vi "main.vi"() -> ()   [LabVIEW 2023]
uses:
  <vilib>/Hampel Software Engineering/Git API/Git API/GIT-api.lvclass
  <vilib>/Utility/miscctls.llb/LVComboBoxStrsAndValuesArrayTypeDef.ctl
  <vilib>/Hampel Software Engineering/Git API/Git API/GIT-api.lvclass/GIT-api.ctl
  <userlib>/_OpenG.lib/file/file.llb/openg_file.lvlib
panel:
  in  "OK":bool
  in  "Repo Url":string="https://github.com/keerthivarman-nageshwaran/LabVIEWGitTool.git"
  in  "Tree":string(tree)
  in  "To":string(combo)
  in  "From":string(combo)
  in  "Diff Tree":string(tree)
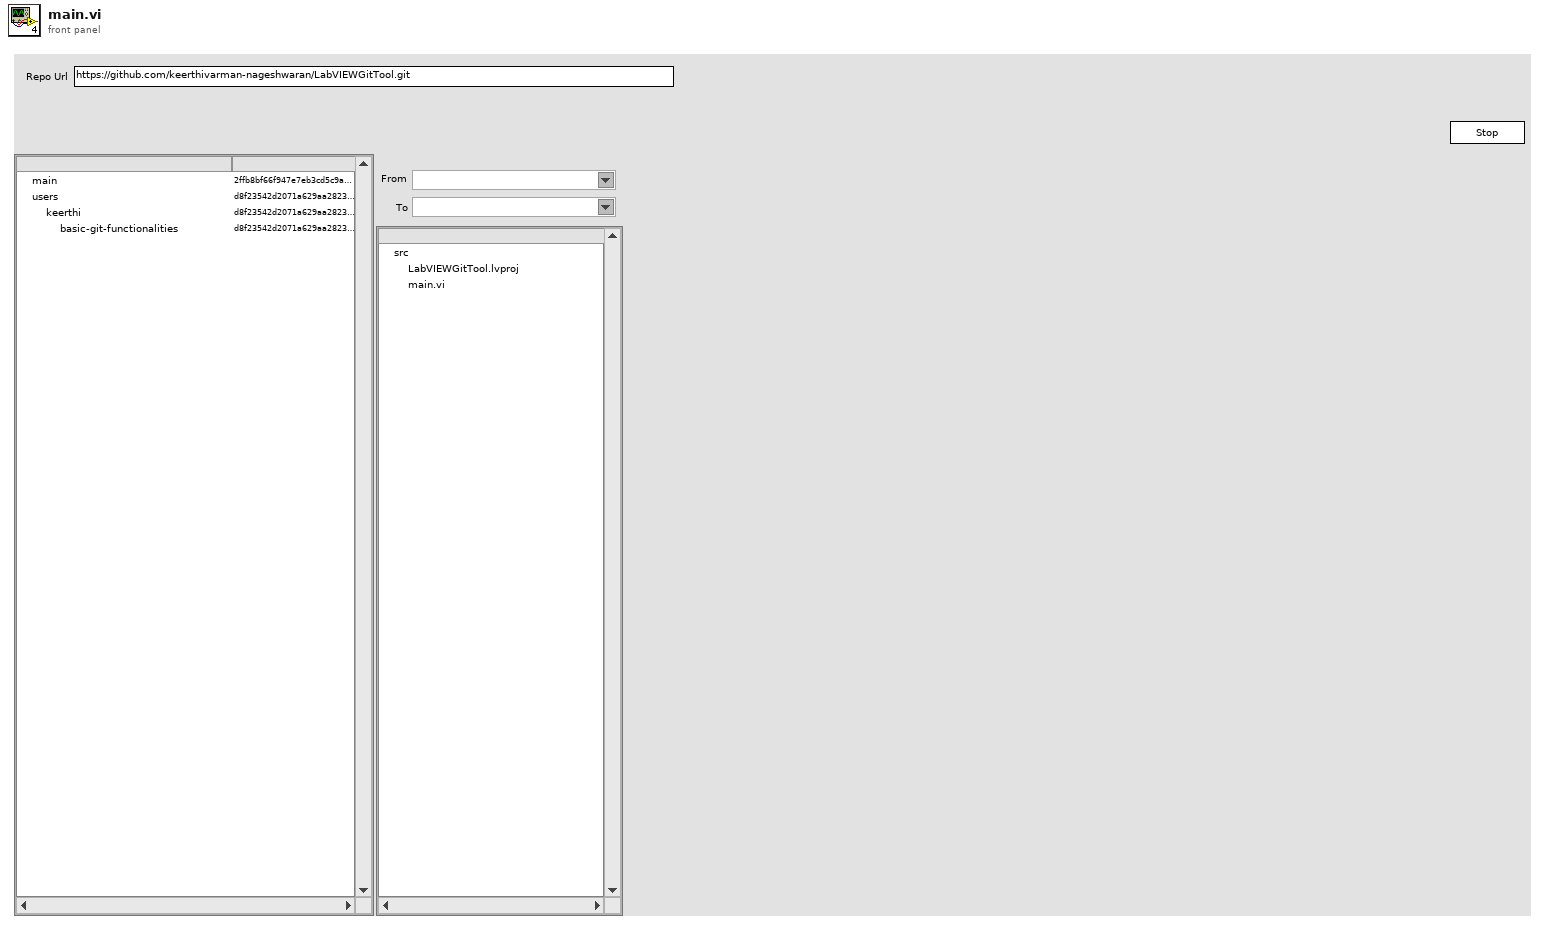
[diagram p1: front panel]
types:
  T1 = cluster{"Core":cluster{"Current VI Reference":refnum<vi>, "Close Panel on Exit?":bool}, "Git":cluster{"Local Repo Path":path, "Repo Url":string, "Temp Path":path, "git-api":refnum<class "GIT-api.lvclass">, "Branches":cluster{"Name":string, "Hash":string}[]}, "UI":cluster{"Tree":refnum<vi>, "Diff Tree":refnum<vi>}, "Diff":cluster{"To":string, "From":string, "Files":string[]}}
  T2 = enum32{"Invalid", "Standard", "Closed", "Hidden", "Minimized", "Maximized"}
  T3 = enum32{"invalid app kind", "Development System", "Run Time System", "Student Edition", "Embedded LabVIEW", "Evaluation", "Custom"}
  T4 = typedef "LVComboBoxStrsAndValuesArrayTypeDef.ctl" = cluster{"String":string, "Value":string}[]
  T5 = cluster{"Current VI Reference":refnum<vi>, "Close Panel on Exit?":bool}
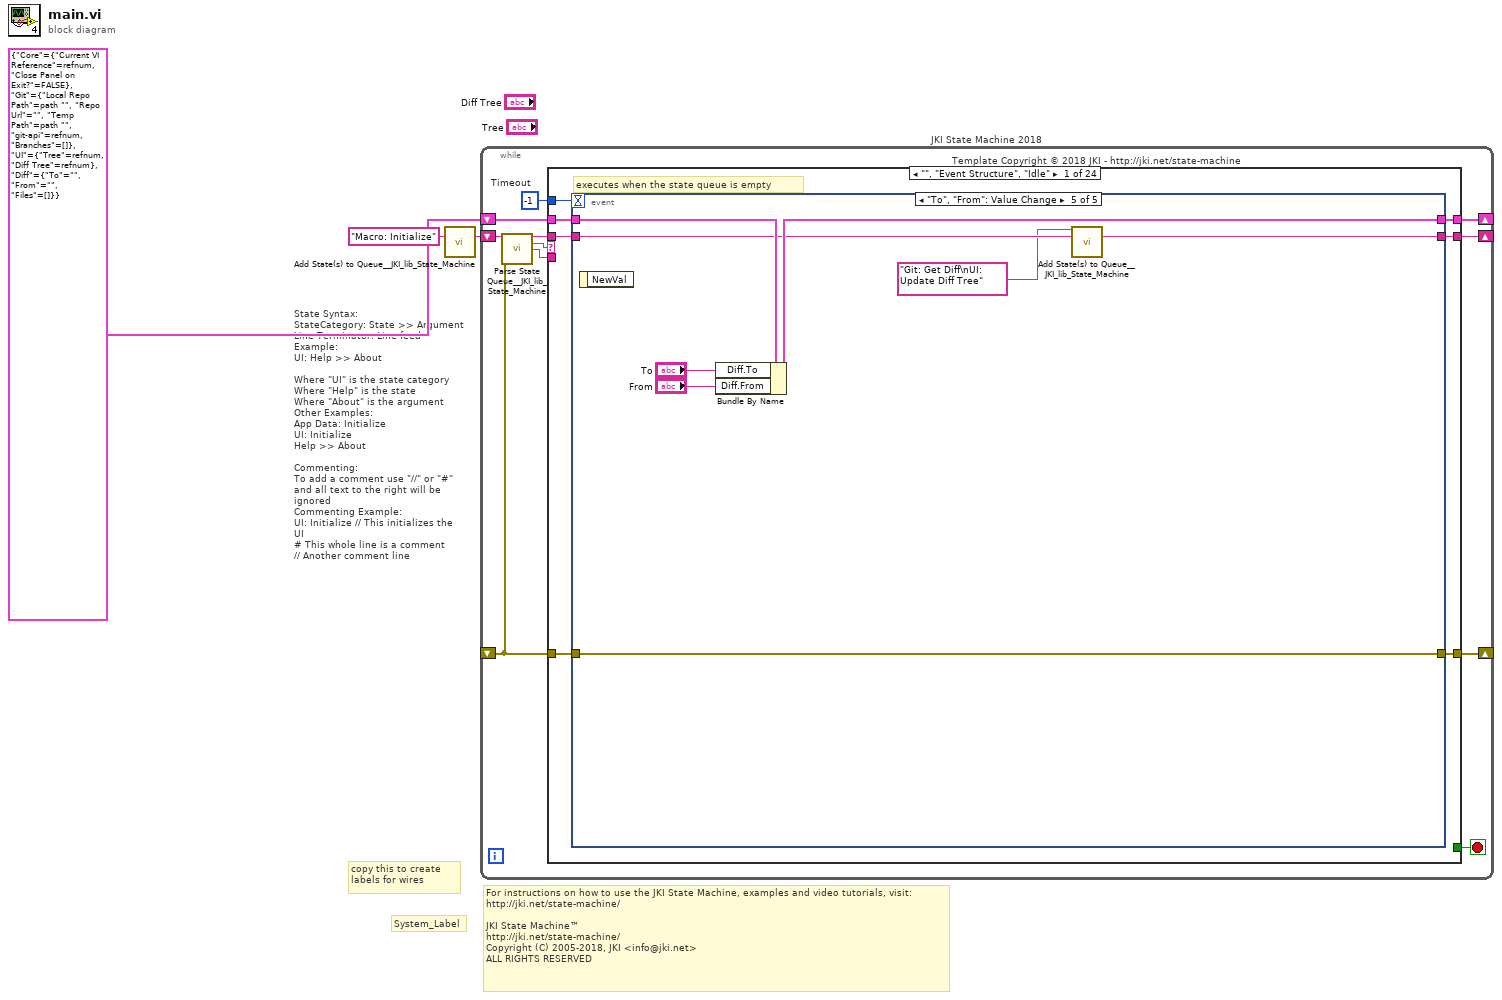
[diagram p0: block diagram]
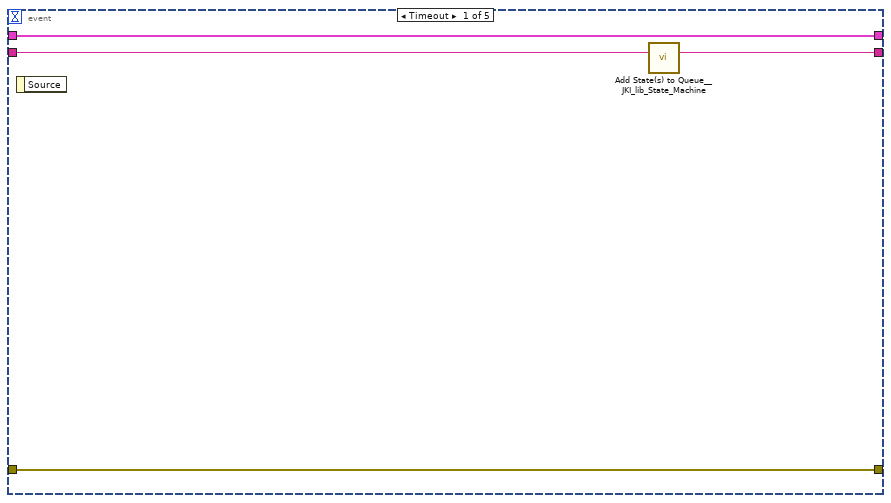
[diagram p2: hidden frame]
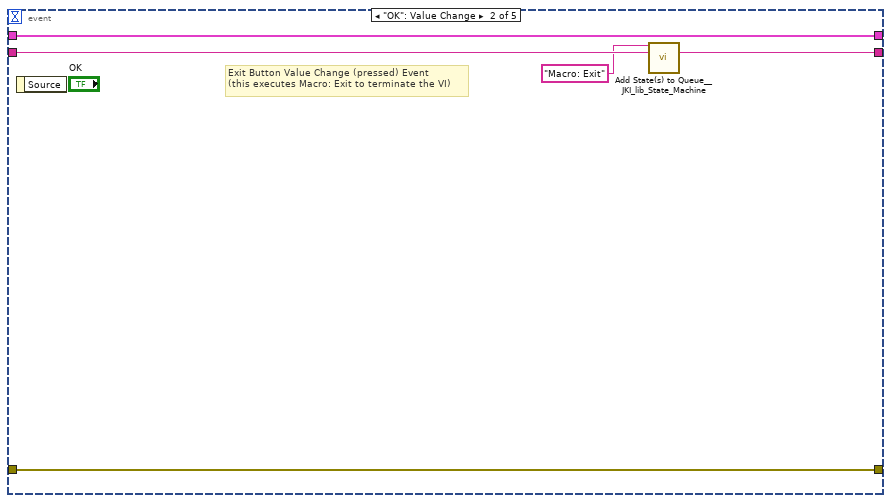
[diagram p3: hidden frame]
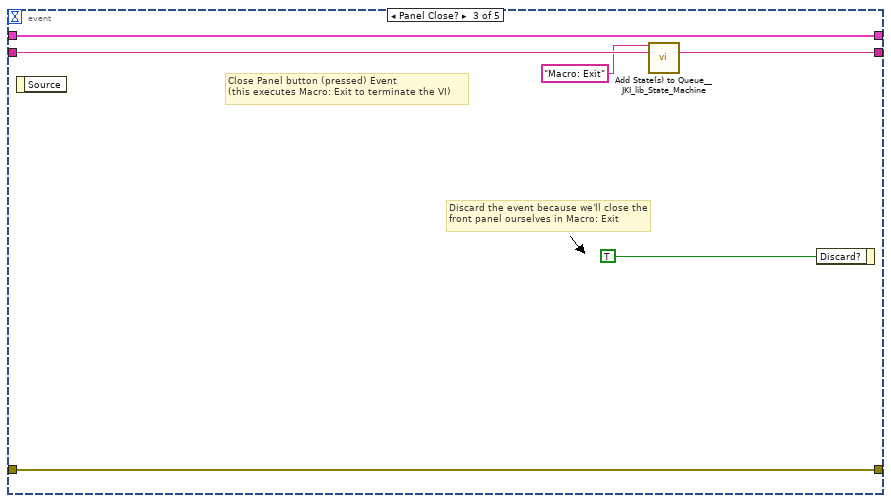
[diagram p4: hidden frame]
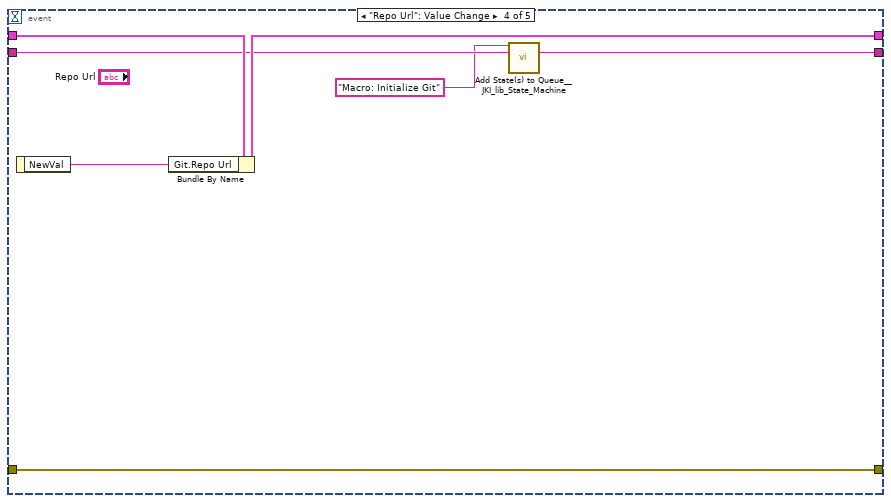
[diagram p5: hidden frame]
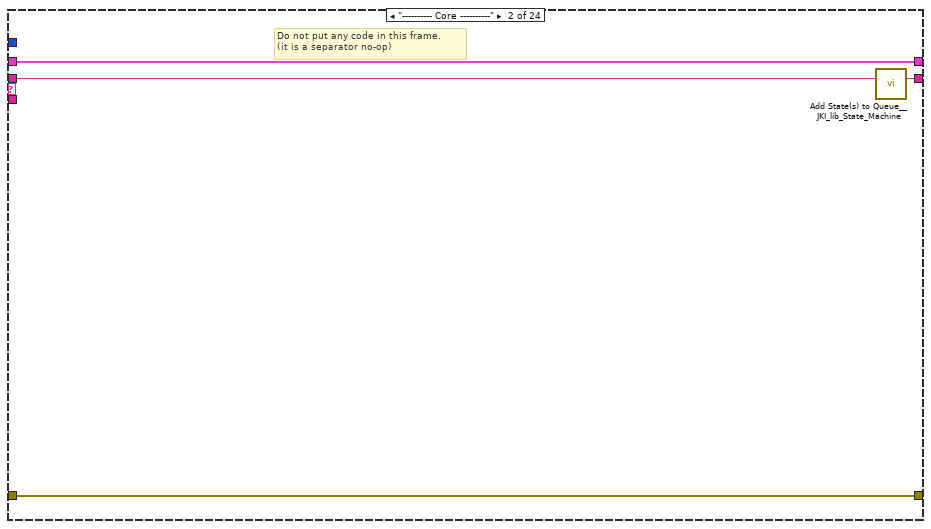
[diagram p6: hidden frame]
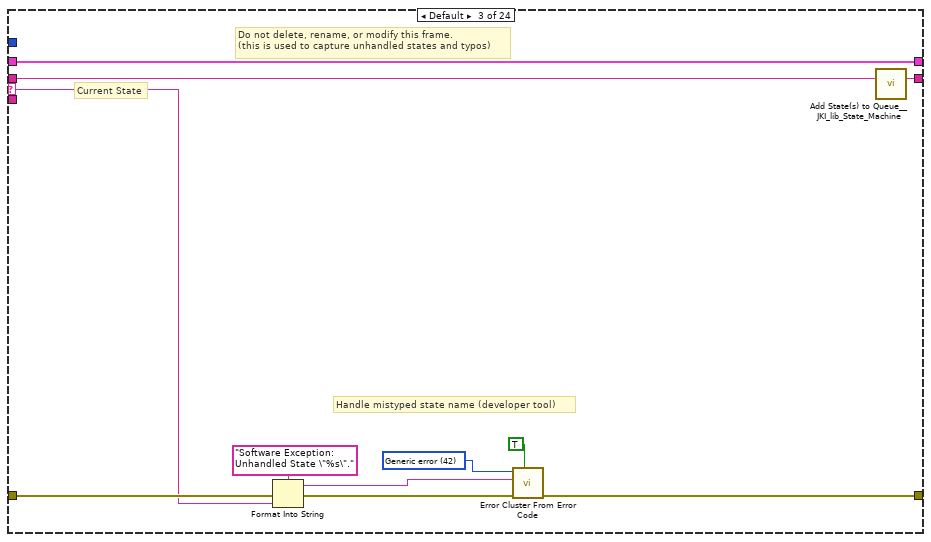
[diagram p7: hidden frame]
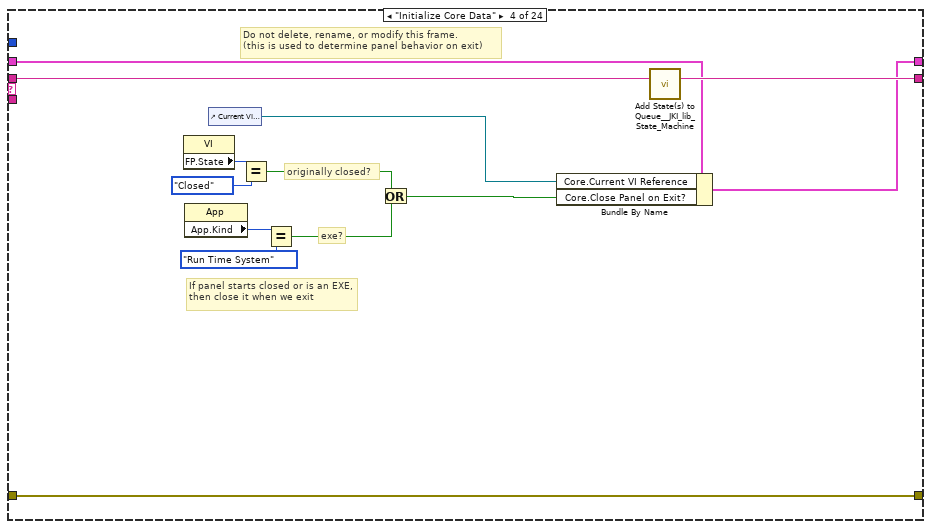
[diagram p8: hidden frame]
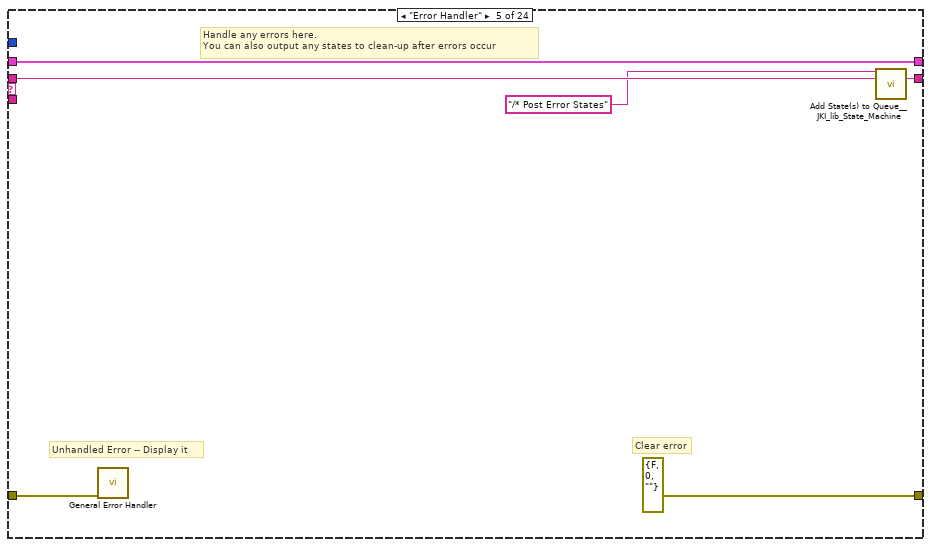
[diagram p9: hidden frame]
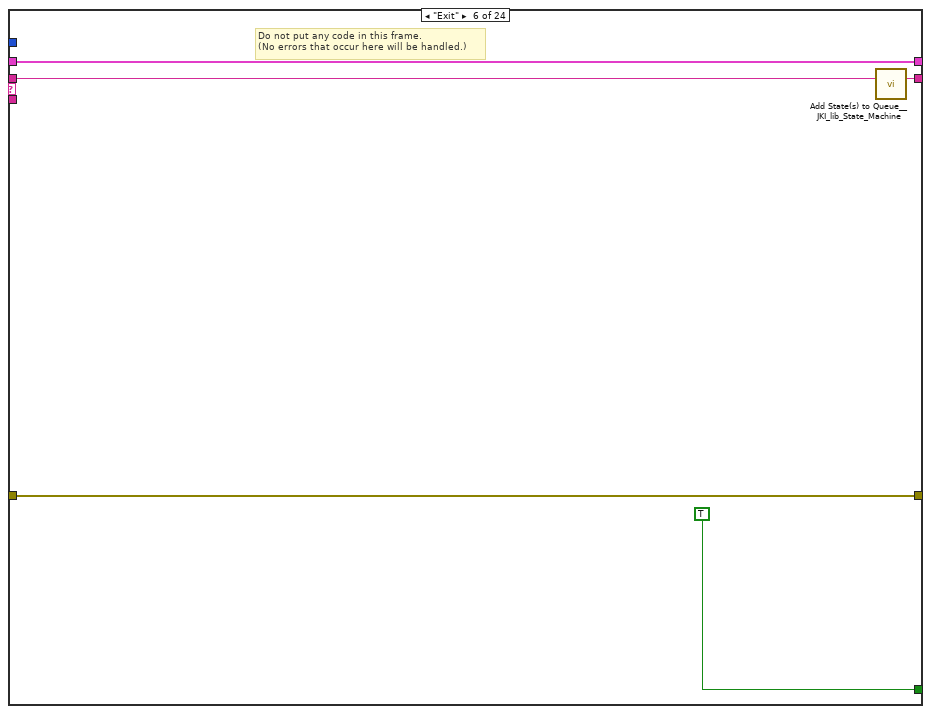
[diagram p10: hidden frame]
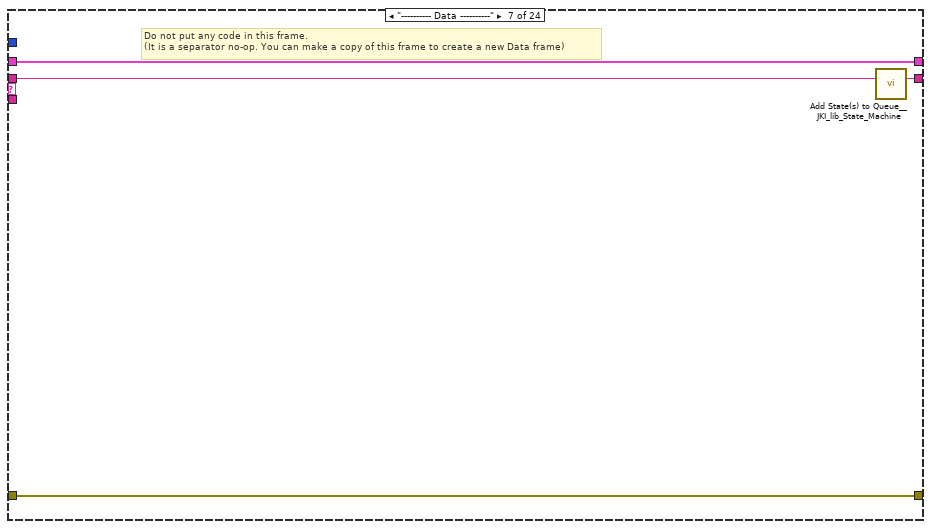
[diagram p11: hidden frame]
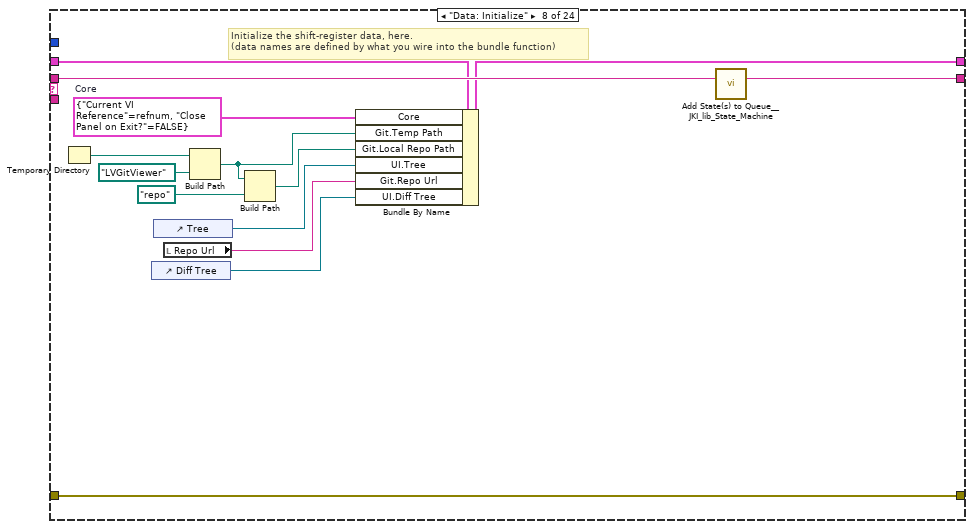
[diagram p12: hidden frame]
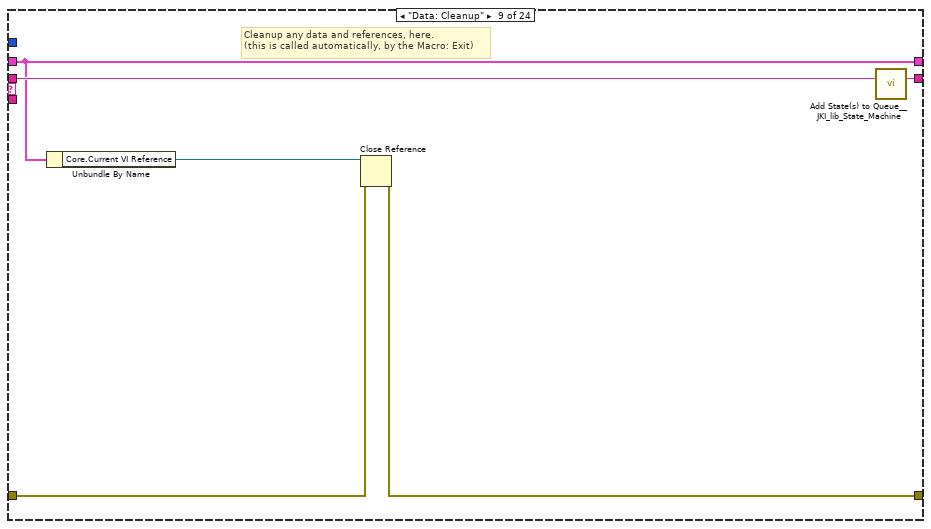
[diagram p13: hidden frame]
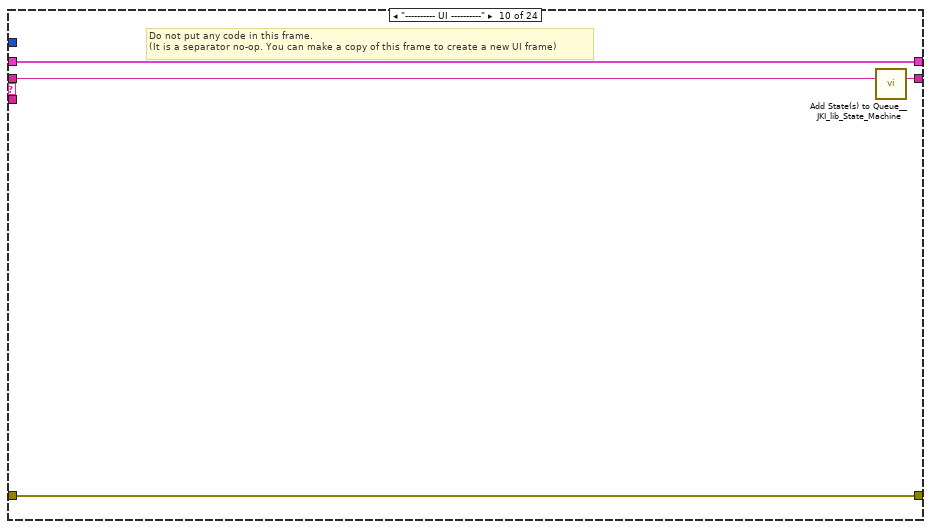
[diagram p14: hidden frame]
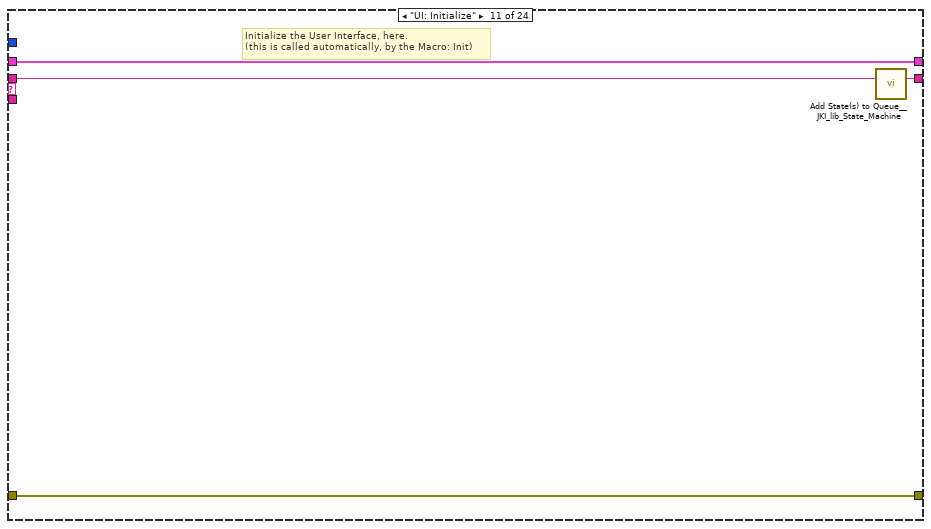
[diagram p15: hidden frame]
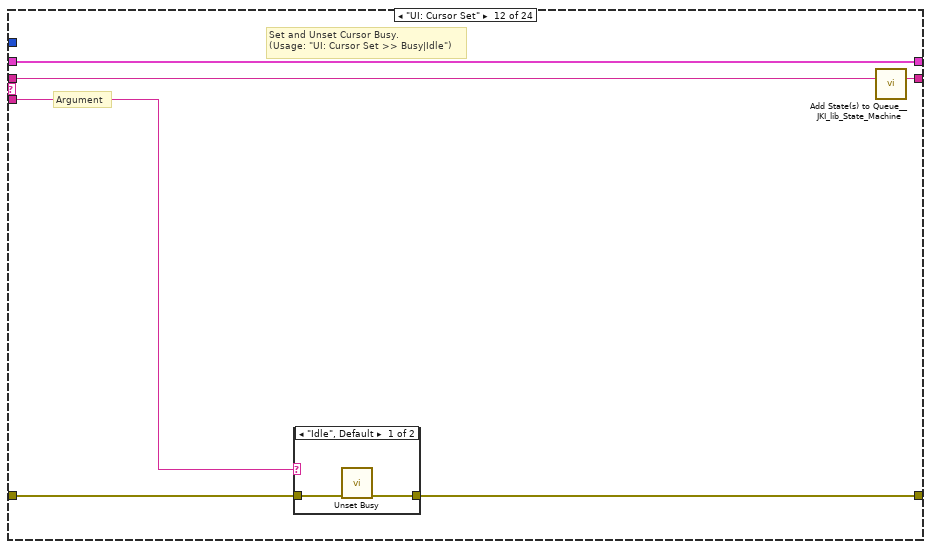
[diagram p16: hidden frame]
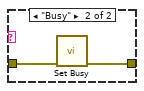
[diagram p17: hidden frame]
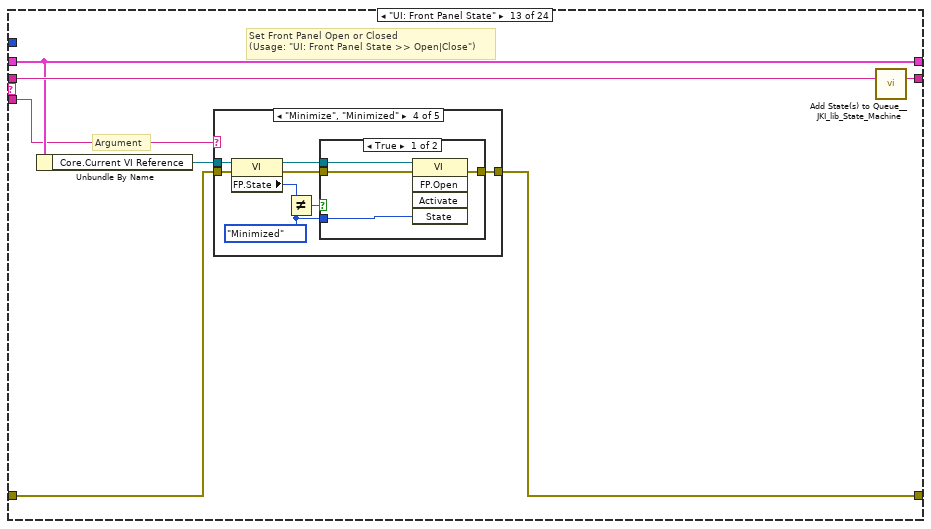
[diagram p18: hidden frame]
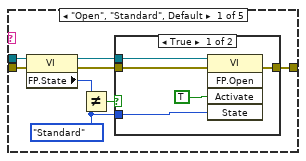
[diagram p19: hidden frame]
diagram:
  # "For instructions on how to use the JKI State Machine, examples and video tutorials, visit:\nhttp://jki.net/state-machine/\n\nJKI State Machine™\nhttp://jki.net/state-machine/\nCopyright (C) 2005-2018, JKI <info@jki.net>\nALL RIGHTS RESERVED"
  # "State Syntax:\nStateCategory: State >> Argument\nLine Terminator: Line feed\nExample:\nUI: Help >> About\n\nWhere \"UI\" is the state category\nWhere \"Help\" is the state\nWhere \"About\" is the argument\nOther Examples:\nApp Data: Initialize\nUI: Initialize\nHelp >> About\n\nCommenting:\nTo add a comment use \"//\" or \"#\" and all text to the right will be ignored\nCommenting Example:\nUI: Initialize // This initializes the UI\n# This whole line is a comment\n// Another comment line"
  # "copy this to create labels for wires"
  # "System_Label"
  n1 = call <vilib>:"Add State(s) to Queue__JKI_lib_State_Machine.vi"("State(s) in (\"\")"="Macro: Initialize") -> ("States Out"=w3:string)  [unwired: 14 in]
  n2 = while "JKI State Machine 2018" {
    shift-right: [w7] -> _
    shift-left: T1 {"Core"={"Current VI Reference"=refnum, "Close Panel on Exit?"=FALSE}, "Git"={"Local Repo Path"=path "", "Repo Url"="", "Temp Path"=path "", "git-api"=refnum, "Branches"=[]}, "UI"={"Tree"=refnum, "Diff Tree"=refnum}, "Diff"={"To"="", "From"="", "Files"=[]}} -> [w6]
    shift-right: [w10] -> _
    shift-left: _ -> [w4]
    shift-right: [w9] -> _
    shift-left: w3 -> [w11]
    stop <- w8 stop-if-true
    w5 = -1  # Timeout
    # "Template Copyright © 2018 JKI - http://jki.net/state-machine"
    n3 = call <vilib>:"Parse State Queue__JKI_lib_State_Machine.vi"("State Queue"=w11, "Error In (no error)"=w4) -> ("Remaining States"=w13:string, "Current State"=w14:string, "Arguments"=w12:string)  [unwired: 11 in]
    n4 = case shown="\"\", \"Event Structure\", \"Idle\"" w14 {
      selector: w14 -> [_ _ w56 _ _ _ _ _ _ _ _ _ _ _ _ _ _ _ _ _ _ _ _ _]
      tunnel: w13 -> [w21 w55 w60 w79 w85 w90 w94 w108 w114 w118 w122 w128 w139 w216 w231 w248 w254 w259 w269 w274 w278 w289 w316 w335]
      tunnel: w12 -> [_ _ _ _ _ _ _ _ _ _ _ w123 w133 _ _ _ _ _ _ _ _ _ _ _]
      tunnel: w6 -> [w19 w52 w58 w72 w82 w88 w91 w104 w109 w115 w120 w126 w135 w212 w229 w244 w251 w256 w266 w271 w275 w287 w314 w333]
      tunnel: [w18 w53 w62 w76 errorcluster {"status"=FALSE, "code"=0, "source"=""} ("error out") w87 w92 w103 w110 w116 w119 w124 w136 w214 w224 w246 w252 w257 w267 w272 w276 w284 w309 w331] -> w10
      tunnel: w4 -> [w17 w53 w61 w76 w81 w87 w92 w103 w111 w116 w119 w125 w137 w213 w223 w245 w252 w257 w267 w272 w276 w282 w310 w328]
      tunnel: [w20 w54 w59 w78 w84 w89 w93 w107 w113 w117 w121 w127 w138 w215 w230 w247 w253 w258 w268 w273 w277 w288 w315 w334] -> w9
      tunnel: [_ _ _ _ _ TRUE _ _ _ _ _ _ _ _ _ _ _ _ _ _ _ _ _ _] -> w8
      tunnel: [w16 w52 w58 w77 w82 w88 w91 w106 w109 w115 w120 w126 w135 w212 w229 w244 w251 w256 w266 w271 w275 w285 w313 w332] -> w7
      tunnel: w5 -> [w15 _ _ _ _ _ _ _ _ _ _ _ _ _ _ _ _ _ _ _ _ _ _ _]
      frame "", "Event Structure", "Idle" {
        # "executes when the state queue is empty"
        n5 = event shown="[4] \"To\", \"From\": Value Change" {
          selector: _ -> [_ _ _ _ _]
          dyn-events: _ -> [_ _ _ _ _]
          timeout: w15 -> [_ _ _ _ _]
          tunnel: w21 -> [w25 w30 w36 w39 w48]
          tunnel: [w24 w29 w35 w38 w47] -> w20
          tunnel: w19 -> [w22 w27 w33 w42 w50]
          tunnel: [w23 w28 w34 w43 w51] -> w18
          tunnel: w17 -> [w23 w28 w34 w43 w51]
          tunnel: [w22 w27 w33 w41 w49] -> w16
          event Timeout {
            n6 = event-data() -> ()  [unwired: 1 in, 1 out]
            n7 = call <vilib>:"Add State(s) to Queue__JKI_lib_State_Machine.vi"("State(s) in (\"\")"=w25) -> ("States Out"=w24:string)  [unwired: 14 in]
          }
          event "OK": Value Change {
            # "Exit Button Value Change (pressed) Event\n(this executes Macro: Exit to terminate the VI)"
            n8 = event-data() -> ()  [unwired: 1 in, 1 out]
            n9 = call <vilib>:"Add State(s) to Queue__JKI_lib_State_Machine.vi"("State(s) in Front (\"\")"="Macro: Exit", "State(s) in (\"\")"=w30) -> ("States Out"=w29:string)  [unwired: 13 in]
          }
          event Panel Close? {
            # "Discard the event because we'll close the front panel ourselves in Macro: Exit"
            # "Close Panel button (pressed) Event\n(this executes Macro: Exit to terminate the VI)"
            n10 = event-data() -> ()  [unwired: 1 in, 1 out]
            n11 = call <vilib>:"Add State(s) to Queue__JKI_lib_State_Machine.vi"("State(s) in Front (\"\")"="Macro: Exit", "State(s) in (\"\")"=w36) -> ("States Out"=w35:string)  [unwired: 13 in]
            n12 = event-data("Discard?"=TRUE) -> ()  [unwired: 1 in, 1 out]
          }
          event "Repo Url": Value Change {
            n13 = event-data() -> ("NewVal"=w40:string)  [unwired: 1 in]
            n14 = Bundle By Name(cluster=w42, "Git.Repo Url"=w40) -> (w41:T1)
            n15 = call <vilib>:"Add State(s) to Queue__JKI_lib_State_Machine.vi"("State(s) in Front (\"\")"="Macro: Initialize Git" ("State(s) in Front (\"\")"), "State(s) in (\"\")"=w39) -> ("States Out"=w38:string)  [unwired: 13 in]
          }
          event "To", "From": Value Change {
            n16 = event-data() -> ()  [unwired: 1 in, 1 out]
            n17 = Bundle By Name(cluster=w50, "Diff.To"="To", "Diff.From"="From") -> (w49:T1)
            n18 = call <vilib>:"Add State(s) to Queue__JKI_lib_State_Machine.vi"("State(s) in Front (\"\")"="Git: Get Diff\nUI: Update Diff Tree" ("State(s) in Front (\"\")"), "State(s) in (\"\")"=w48) -> ("States Out"=w47:string)  [unwired: 13 in]
          }
        }
      }
      frame "---------- Core ----------" {
        # "Do not put any code in this frame.\n(it is a separator no-op)"
        n19 = call <vilib>:"Add State(s) to Queue__JKI_lib_State_Machine.vi"("State(s) in (\"\")"=w55) -> ("States Out"=w54:string)  [unwired: 14 in]
      }
      frame Default {
        w65 = 42 items=["No error", "Argument error", "Memory is full", "Out of zone", "End of file", "File already open", "Generic file I/O error", "File not found", "File permission error", "Disk is full", "Duplicate path", "Too many files open", "System feature not enabled", "Resource file not found", "Cannot add resource", "Resource not found", "Image not found", "Image memory error", "Pen does not exist", "Config type invalid", "Config token not found", "Config parse error", "Config memory error", "Bad external code format", "Bad external code offset", "External code not present", "Null window", "Destroy window error", "Null menu", "Print aborted", "Bad print record", "Print driver error", "Windows error during printing", "Memory error during printing", "Print dialog error", "Generic print error", "Invalid device refnum", "Device not found", "Device parameter error", "Device unit error", "Cannot open device", "Device call aborted", "Generic error", "Cancelled by user", "Object ID too low", "Object ID too high", "Object not in heap", "Unknown heap", "Unknown object (invalid DefProc)", "Unknown object (DefProc not in table)", "Message out of range", "Invalid (null) method", "Unknown message", "Manager call not supported", "Bad address", "Network operation in progress", "Network operation timed out", "Connection is busy", "Network attribute not supported", "Network error", "Address in use", "System out of memory", "Connection aborted", "Connection refused", "Not connected", "Already connected", "Connection closed", "Initialization error (interapplication manager)", "Bad occurrence", "Wait on unbound occurrence handler", "Occurrence queue overflow", "Datalog type conflict", "Unused", "Unrecognized type (interapplication manager)", "Memory corrupt", "Failed to make temporary DLL", "Old CIN version", "Drag socket not found", "Failed to load drop-object", "Failed to register OLE object", "Failed to release OLE object", "Format specifier type mismatch", "Unknown format specifier", "Too few format specifiers", "Too many format specifiers", "Scan failed", "Newer CIN version", "Error converting to variant", "Runtime menu error", "Password tampered", "Variant attribute not found", "Incompatible variant data type", "Event data is not available", "Event Store is not present", "Occurrence is not found", "Event Queue is not created", "Event info is not available", "Refnum passed is NULL", "Error retrieving Class GUID", "Error retrieving CoClass GUID", "Error retrieving TypeLib GUID.", "Bad built application magic bytes.", "Specific driver is different from the specific driver associated with the Logical Name.", "There is no session opened to the class driver.", "Max Error", "MAX - Error with config objects", "MAX - Error loading configuration", "MAX - Group not supported"]
        # "Current State"
        # "Do not delete, rename, or modify this frame.\n(this is used to capture unhandled states and typos)"
        # "Handle mistyped state name (developer tool)"
        n20 = Format Into String(format string="Software Exception: Unhandled State \"%s\"." ("message"), error in=w61, w56) -> (resulting string=w64:string, error out=w63:errorcluster)  [unwired: 1 in]
        n21 = call <vilib>:"Error Cluster From Error Code.vi"("show call chain? (False)"=TRUE, "error in (no error)"=w63, "error message (\"\")"=w64, "error code (0)"=w65) -> ("error out"=w62:errorcluster)  [unwired: 5 in]
        n22 = call <vilib>:"Add State(s) to Queue__JKI_lib_State_Machine.vi"("State(s) in (\"\")"=w60) -> ("States Out"=w59:string)  [unwired: 14 in]
      }
      frame "Initialize Core Data" {
        # "Do not delete, rename, or modify this frame.\n(this is used to determine panel behavior on exit)"
        # "originally closed?"
        # "exe?"
        # "If panel starts closed or is an EXE, then close it when we exit"
        n23 = property class="VI"() -> ("FP.State"=w69:T2)  [unwired: 2 in, 2 out]
        n24 = property class="App"() -> ("App.Kind"=w75:T3)  [unwired: 2 in, 2 out]
        n25 = control-ref of="Current VI Reference"() -> (w70:refnum<vi>)
        n26 = Equal?(x=w69, y=T2."Closed" ("Front Panel Window:State")) -> (x = y?=w67:bool)
        n27 = Equal?(x=w75, y=T3."Run Time System" ("Application:Kind")) -> (x = y?=w73:bool)
        n28 = Or(x=w67, y=w73) -> (x .or. y?=w71:bool)
        n29 = Bundle By Name(cluster=w72, "Core.Current VI Reference"=w70, "Core.Close Panel on Exit?"=w71) -> (w77:T1)
        n30 = call <vilib>:"Add State(s) to Queue__JKI_lib_State_Machine.vi"("State(s) in (\"\")"=w79) -> ("States Out"=w78:string)  [unwired: 14 in]
      }
      frame "Error Handler" {
        # "Unhandled Error -- Display it"
        # "Handle any errors here.\nYou can also output any states to clean-up after errors occur"
        # "Clear error"
        n31 = call <vilib>:"General Error Handler.vi"("error in (no error)"=w81) -> ()  [unwired: 10 in, 5 out]
        n32 = call <vilib>:"Add State(s) to Queue__JKI_lib_State_Machine.vi"("State(s) in Front (\"\")"="/* Post Error States", "State(s) in (\"\")"=w85) -> ("States Out"=w84:string)  [unwired: 13 in]
      }
      frame "Exit" {
        # "Do not put any code in this frame.\n(No errors that occur here will be handled.)"
        n33 = call <vilib>:"Add State(s) to Queue__JKI_lib_State_Machine.vi"("State(s) in (\"\")"=w90) -> ("States Out"=w89:string)  [unwired: 14 in]
      }
      frame "---------- Data ----------" {
        # "Do not put any code in this frame.\n(It is a separator no-op. You can make a copy of this frame to create a new Data frame)"
        n34 = call <vilib>:"Add State(s) to Queue__JKI_lib_State_Machine.vi"("State(s) in (\"\")"=w94) -> ("States Out"=w93:string)  [unwired: 14 in]
      }
      frame "Data: Initialize" {
        w105 = T5 {"Current VI Reference"=refnum, "Close Panel on Exit?"=FALSE}  # Core
        # "Initialize the shift-register data, here.\n(data names are defined by what you wire into the bundle function)"
        n35 = Temporary Directory() -> (w102:path)
        n36 = control-ref of="Diff Tree"() -> (w95:refnum<vi>)
        n37 = control-ref of="Tree"() -> (w97:refnum<vi>)
        n38 = local read "Repo Url"() -> (w96:string)
        n39 = Build Path(base path=w102, name or relative path=path "LVGitViewer") -> (appended path=w100:path)
        n40 = Build Path(base path=w100, name or relative path=path "repo") -> (appended path=w99:path)
        n41 = Bundle By Name(cluster=w104, "Core"=w105, "Git.Temp Path"=w100, "Git.Local Repo Path"=w99, "UI.Tree"=w97, "Git.Repo Url"=w96, "UI.Diff Tree"=w95) -> (w106:T1)
        n42 = call <vilib>:"Add State(s) to Queue__JKI_lib_State_Machine.vi"("State(s) in (\"\")"=w108) -> ("States Out"=w107:string)  [unwired: 14 in]
      }
      frame "Data: Cleanup" {
        # "Cleanup any data and references, here.\n(this is called automatically, by the Macro: Exit)"
        n43 = Unbundle By Name(w109) -> ("Core.Current VI Reference"=w112:refnum<vi>)
        n44 = Close Reference(reference=w112, error in (no error)=w111) -> (error out=w110:errorcluster)
        n45 = call <vilib>:"Add State(s) to Queue__JKI_lib_State_Machine.vi"("State(s) in (\"\")"=w114) -> ("States Out"=w113:string)  [unwired: 14 in]
      }
      frame "---------- UI ----------" {
        # "Do not put any code in this frame.\n(It is a separator no-op. You can make a copy of this frame to create a new UI frame)"
        n46 = call <vilib>:"Add State(s) to Queue__JKI_lib_State_Machine.vi"("State(s) in (\"\")"=w118) -> ("States Out"=w117:string)  [unwired: 14 in]
      }
      frame "UI: Initialize" {
        # "Initialize the User Interface, here.\n(this is called automatically, by the Macro: Init)"
        n47 = call <vilib>:"Add State(s) to Queue__JKI_lib_State_Machine.vi"("State(s) in (\"\")"=w122) -> ("States Out"=w121:string)  [unwired: 14 in]
      }
      frame "UI: Cursor Set" {
        # "Argument"
        # "Set and Unset Cursor Busy.\n(Usage: \"UI: Cursor Set >> Busy|Idle\")"
        n48 = case shown="\"Idle\", Default" w123 {
          tunnel: w125 -> [w130 w132]
          tunnel: [w129 w131] -> w124
          frame "Idle", Default {
            n49 = call <vilib>:"Unset Busy.vi"("error in (no error)"=w130) -> ("error out"=w129:errorcluster)  [unwired: 10 in]
          }
          frame "Busy" {
            n50 = call <vilib>:"Set Busy.vi"("error in (no error)"=w132) -> ("error out"=w131:errorcluster)  [unwired: 9 in, 1 out]
          }
        }
        n51 = call <vilib>:"Add State(s) to Queue__JKI_lib_State_Machine.vi"("State(s) in (\"\")"=w128) -> ("States Out"=w127:string)  [unwired: 14 in]
      }
      frame "UI: Front Panel State" {
        # "Argument"
        # "Set Front Panel Open or Closed\n(Usage: \"UI: Front Panel State >> Open|Close\")"
        n52 = Unbundle By Name(w135) -> ("Core.Current VI Reference"=w134:refnum<vi>)
        n53 = case shown="\"Minimize\", \"Minimized\"" w133 {
          tunnel: w137 -> [w145 w160 w171 w184 w197]
          tunnel: [w147 w161 w173 w186 w199] -> w136
          tunnel: w134 -> [w146 w158 w172 w185 w198]
          frame "Open", "Standard", Default {
            w140 = T2."Standard" ("State")
            n54 = property class="VI"(reference=w146, error in=w145) -> (reference out=w143:refnum<vi>, error out=w144:errorcluster, "FP.State"=w142:T2)
            n55 = Not Equal?(x=w142, y=w140) -> (x != y?=w141:bool)
            n56 = case shown="True" w141 {
              tunnel: [w151 w153] -> w147
              tunnel: w144 -> [w150 w153]
              tunnel: w143 -> [w149 _]
              tunnel: w140 -> [w148 _]
              frame True {
                n57 = invoke class="VI" method="FP.Open"(reference=w149, error in=w150, "Activate"=TRUE, "State"=w148) -> (error out=w151:errorcluster)  [unwired: 1 in, 4 out]
              }
              frame False {
              }
            }
          }
          frame "Close", "Closed" {
            n58 = property class="VI"(reference=w158, error in=w160) -> (reference out=w157:refnum<vi>, error out=w159:errorcluster, "FP.State"=w155:T2)
            n59 = Not Equal?(x=w155, y=T2."Closed" ("Front Panel Window:State")) -> (x != y?=w154:bool)
            n60 = case shown="True" w154 {
              tunnel: [w162 w165] -> w161
              tunnel: w159 -> [w162 w164]
              tunnel: w157 -> [_ w163]
              frame False {
              }
              frame True {
                n61 = invoke class="VI" method="FP.Close"(reference=w163, error in=w164) -> (error out=w165:errorcluster)  [unwired: 1 in, 2 out]
              }
            }
          }
          frame "Hidden", "Hide" {
            w166 = T2."Hidden" ("State")
            n62 = property class="VI"(reference=w172, error in=w171) -> (reference out=w169:refnum<vi>, error out=w170:errorcluster, "FP.State"=w168:T2)
            n63 = Not Equal?(x=w168, y=w166) -> (x != y?=w167:bool)
            n64 = case shown="True" w167 {
              tunnel: [w177 w178] -> w173
              tunnel: w170 -> [w176 w178]
              tunnel: w169 -> [w175 _]
              tunnel: w166 -> [w174 _]
              frame True {
                n65 = invoke class="VI" method="FP.Open"(reference=w175, error in=w176, "State"=w174) -> (error out=w177:errorcluster)  [unwired: 2 in, 4 out]
              }
              frame False {
              }
            }
          }
          frame "Minimize", "Minimized" {
            w179 = T2."Minimized" ("State")
            n66 = property class="VI"(reference=w185, error in=w184) -> (reference out=w182:refnum<vi>, error out=w183:errorcluster, "FP.State"=w181:T2)
            n67 = Not Equal?(x=w181, y=w179) -> (x != y?=w180:bool)
            n68 = case shown="True" w180 {
              tunnel: [w190 w191] -> w186
              tunnel: w183 -> [w189 w191]
              tunnel: w182 -> [w188 _]
              tunnel: w179 -> [w187 _]
              frame True {
                n69 = invoke class="VI" method="FP.Open"(reference=w188, error in=w189, "State"=w187) -> (error out=w190:errorcluster)  [unwired: 2 in, 4 out]
              }
              frame False {
              }
            }
          }
          frame "Maximize", "Maximized" {
            w192 = T2."Maximized" ("State")
            n70 = property class="VI"(reference=w198, error in=w197) -> (reference out=w195:refnum<vi>, error out=w196:errorcluster, "FP.State"=w194:T2)
            n71 = Not Equal?(x=w194, y=w192) -> (x != y?=w193:bool)
            n72 = case shown="True" w193 {
              tunnel: [w203 w204] -> w199
              tunnel: w196 -> [w202 w204]
              tunnel: w195 -> [w201 _]
              tunnel: w192 -> [w200 _]
              frame True {
                n73 = invoke class="VI" method="FP.Open"(reference=w201, error in=w202, "State"=w200) -> (error out=w203:errorcluster)  [unwired: 2 in, 4 out]
              }
              frame False {
              }
            }
          }
        }
        n74 = call <vilib>:"Add State(s) to Queue__JKI_lib_State_Machine.vi"("State(s) in (\"\")"=w139) -> ("States Out"=w138:string)  [unwired: 14 in]
      }
      frame "UI: Update Branches" {
        n75 = Unbundle By Name(w212) -> ("UI.Tree"=w211:refnum<vi>, "Git.Branches"=w209:cluster{"Name":string, "Hash":string}[])
        n76 = for {
          tunnel: w209 -> [w220] mode=indexing
          tunnel: [w217] -> w208 mode=indexing
          n77 = Unbundle By Name(w220) -> ("Name"=w219:string, "Hash"=w218:string)
          n78 = Build Array(w219, w218) -> (w217:string[])
        }
        n79 = call <userlib>:"MGI Populate Tree with Delimited Strings.vi"("Use Child Only?"=TRUE, "Default Symbol"=0, "error in (no error)"=w213, "Delimiter"="/", "Items (Delimited)"=w208, "Tree Control"=w211) -> ("error out"=w214:errorcluster)  [unwired: 3 in, 2 out]
        n80 = call <vilib>:"Add State(s) to Queue__JKI_lib_State_Machine.vi"("State(s) in Front (\"\")"="UI: Update Branches 1" ("State(s) in Front (\"\")"), "State(s) in (\"\")"=w216) -> ("States Out"=w215:string)  [unwired: 13 in]
      }
      frame "UI: Update Branches 1" {
        n81 = Unbundle By Name(w229) -> ("Git.Branches"=w228:cluster{"Name":string, "Hash":string}[])
        n82 = Index Array(array=T4 [] ("Strings And Values []")) -> (element=w226:cluster{"String":string, "Value":string})  [unwired: 1 in]
        n83 = for {
          tunnel: w228 -> [w236] mode=indexing
          tunnel: w226 -> [w235]
          tunnel: [w234] -> w225 mode=indexing
          n84 = Unbundle By Name(w236) -> ("Name"=w232:string, "Hash"=w233:string)
          n85 = Bundle By Name(cluster=w235, "String"=w232, "Value"=w233) -> (w234:cluster{"String":string, "Value":string})
        }
        n86 = property on="From" class="CmbBox"("Strings And Values[]"=w225) -> (error out=w222:errorcluster)  [unwired: 2 in, 1 out]
        n87 = property on="To" class="CmbBox"("Strings And Values[]"=w225) -> (error out=w221:errorcluster)  [unwired: 2 in, 1 out]
        n88 = Merge Errors(w222, w221, w223) -> (w224:errorcluster)
        n89 = call <vilib>:"Add State(s) to Queue__JKI_lib_State_Machine.vi"("State(s) in (\"\")"=w231) -> ("States Out"=w230:string)  [unwired: 14 in]
      }
      frame "UI: Update Diff Tree" {
        n90 = Unbundle By Name(w244) -> ("UI.Diff Tree"=w243:refnum<vi>, "Diff.Files"=w241:string[])
        n91 = for {
          tunnel: w241 -> [w249] mode=indexing
          tunnel: [w250] -> w240 mode=indexing
          n92 = Build Array(w249) -> (w250:string[])
        }
        n93 = call <userlib>:"MGI Populate Tree with Delimited Strings.vi"("Use Child Only?"=TRUE, "Default Symbol"=0, "error in (no error)"=w245, "Delimiter"="/", "Items (Delimited)"=w240, "Tree Control"=w243) -> ("error out"=w246:errorcluster)  [unwired: 3 in, 2 out]
        n94 = call <vilib>:"Add State(s) to Queue__JKI_lib_State_Machine.vi"("State(s) in Front (\"\")"="UI: Update Branches 1" ("State(s) in Front (\"\")"), "State(s) in (\"\")"=w248) -> ("States Out"=w247:string)  [unwired: 13 in]
      }
      frame "---------- Macro ----------" {
        # "Do not put any code in this frame.\n(It is a separator no-op. You can make a copy of this frame to create a new Macro frame)"
        n95 = call <vilib>:"Add State(s) to Queue__JKI_lib_State_Machine.vi"("State(s) in (\"\")"=w254) -> ("States Out"=w253:string)  [unwired: 14 in]
      }
      frame "Macro: Initialize" {
        # "Initialization Macro\n(This is called once, when the VI starts)"
        n96 = call <vilib>:"Add State(s) to Queue__JKI_lib_State_Machine.vi"("State(s) in Front (\"\")"="Data: Initialize\nInitialize Core Data\nUI: Initialize\nMacro: Initialize Git\nUI: Front Panel State >> Open", "State(s) in (\"\")"=w259) -> ("States Out"=w258:string)  [unwired: 13 in]
      }
      frame "Macro: Exit" {
        # "Exit Macro\n(This is called once, when the VI exits)"
        n97 = Unbundle By Name(w266) -> ("Core.Close Panel on Exit?"=w265:bool)
        n98 = Select(t="UI: Front Panel State >> Close", s=w265, f="") -> (s? t:f=w262:string)
        n99 = call <vilib>:"Add State(s) to Queue__JKI_lib_State_Machine.vi"("State(s) in (\"\")"=w262, "State(s) at Back (\"\")"="Data: Cleanup\nExit") -> ("States Out"=w260:string)  [unwired: 13 in]
        n100 = call <vilib>:"Add State(s) to Queue__JKI_lib_State_Machine.vi"("State(s) in Front (\"\")"=w260, "State(s) in (\"\")"=w269) -> ("States Out"=w268:string)  [unwired: 13 in]
      }
      frame "Macro: Initialize Git" {
        # "Initialization Macro\n(This is called once, when the VI starts)"
        n101 = call <vilib>:"Add State(s) to Queue__JKI_lib_State_Machine.vi"("State(s) in Front (\"\")"="Git: Initialize\nGit: Get Branches\nUI: Update Branches", "State(s) in (\"\")"=w274) -> ("States Out"=w273:string)  [unwired: 13 in]
      }
      frame "---------- Git ----------" {
        # "Template Separator\n(You can make a copy of, or modify, this frame)"
        n102 = call <vilib>:"Add State(s) to Queue__JKI_lib_State_Machine.vi"("State(s) in (\"\")"=w278) -> ("States Out"=w277:string)  [unwired: 14 in]
      }
      frame "Git: Initialize" {
        n103 = Unbundle By Name(w287) -> ("Git.Local Repo Path"=w286:path, "Git.Repo Url"=w280:string, "Git.Local Repo Path"=w281:path)
        n104 = Empty String/Path?(string/path=w280) -> (empty?=w279:bool)
        n105 = case "Empty Repo URL?" shown="False" w279 {
          tunnel: w280 -> [w298 _]
          tunnel: w286 -> [w297 _]
          tunnel: [w296 w304] -> w284
          tunnel: [w295 refnum<class "GIT-api.lvclass"> refnum ("git-api out")] -> w283
          tunnel: w282 -> [w293 w304]
          tunnel: w281 -> [w292 _]
          frame False {
            n106 = call <userlib>:"Delete Recursive__ogtk.vi"("error in (no error)"=w293, "Ignore Read-Only? (FALSE)"=TRUE, "Recursive? (FALSE)"=TRUE, "Path"=w292) -> ("error out"=w294:errorcluster)  [unwired: 6 in, 1 out]
            n107 = call <vilib>:"GIT-Create API.vi"("error in"=w294) -> ("error out"=w300:errorcluster, "git-api out"=w299:refnum<class "GIT-api.lvclass">)  [unwired: 9 in]
            n108 = call <vilib>:"GIT-Clone.vi"("error in"=w300, "Local Path"=w292, "Repository URL"=w298, "git-api in"=w299) -> ("error out"=w302:errorcluster, "git-api out"=w301:refnum<class "GIT-api.lvclass">)  [unwired: 5 in, 1 out]
            n109 = call <vilib>:"GIT-Set Working Dir.vi"("error in"=w302, "Working Directory"=w297, "git-api in"=w301) -> ("error out"=w296:errorcluster, "git-api out"=w295:refnum<class "GIT-api.lvclass">)  [unwired: 7 in]
          }
          frame True {
          }
        }
        n110 = Bundle By Name(cluster=w287, "Git.git-api"=w283) -> (w285:T1)
        n111 = call <vilib>:"Add State(s) to Queue__JKI_lib_State_Machine.vi"("State(s) in (\"\")"=w289) -> ("States Out"=w288:string)  [unwired: 14 in]
      }
      frame "Git: Get Branches" {
        n112 = Unbundle By Name(w314) -> ("Git.Branches"=w308:cluster{"Name":string, "Hash":string}[], "Git.git-api"=w312:refnum<class "GIT-api.lvclass">)
        n113 = call <vilib>:"GIT-Remote Branches.vi"("error in"=w310, "git-api in"=w312) -> ("error out"=w309:errorcluster, "branches"=w306:string[][], "git-api out"=w311:refnum<class "GIT-api.lvclass">)  [unwired: 7 in]
        n114 = Index Array(array=w308) -> (element=w307:cluster{"Name":string, "Hash":string})  [unwired: 1 in]
        n115 = for {
          tunnel: w307 -> [w321]
          tunnel: [w320] -> w305 mode=indexing
          tunnel: w306 -> [w319] mode=indexing
          n116 = Index Array(array=w319) -> (element #1=w318:string, element #2=w317:string)  [unwired: 2 in]
          n117 = Bundle By Name(cluster=w321, "Hash"=w318, "Name"=w317) -> (w320:cluster{"Name":string, "Hash":string})
        }
        n118 = Bundle By Name(cluster=w314, "Git.Branches"=w305, "Git.git-api"=w311) -> (w313:T1)
        n119 = call <vilib>:"Add State(s) to Queue__JKI_lib_State_Machine.vi"("State(s) in (\"\")"=w316) -> ("States Out"=w315:string)  [unwired: 14 in]
      }
      frame "Git: Get Diff" {
        n120 = Unbundle By Name(w333) -> ("Diff.From"=w326:string, "Diff.To"=w325:string, "Git.git-api"=w330:refnum<class "GIT-api.lvclass">)
        n121 = Empty String/Path?(string/path=w326) -> (empty?=w324:bool)
        n122 = Empty String/Path?(string/path=w325) -> (empty?=w323:bool)
        n123 = Compound Arithmetic op=OR(w324, w323) -> (w322:bool)
        n124 = case "Any Empty Branch?" shown="False" w322 {
          tunnel: [w349 w352] -> w331
          tunnel: w330 -> [w348 w351]
          tunnel: [w347 w351] -> w329
          tunnel: w328 -> [w343 w352]
          tunnel: w326 -> [w342 _]
          tunnel: w325 -> [w341 _]
          tunnel: [w337 string[] [] ("format string")] -> w327
          frame False {
            # "git diff --name-only <branch_1>..<branch_2>"
            n125 = Format Into String(format string="diff --name-only %s..%s", error in=w343, w342, w341) -> (resulting string=w345:string, error out=w344:errorcluster)  [unwired: 1 in]
            n126 = call <vilib>:"GIT-Execute Cmd.vi"("Command"=w345, "error in"=w344, "Git-API in"=w348) -> ("error out"=w349:errorcluster, "Git-API out"=w347:refnum<class "GIT-api.lvclass">, "std out"=w340:string)  [unwired: 6 in]
            n127 = Spreadsheet String To Array(delimiter (Tab)="\n", format string="", spreadsheet string=w340, array type (2D Dbl)=string[] [] ("format string")) -> (array=w337:string[])
          }
          frame True {
          }
        }
        n128 = Bundle By Name(cluster=w333, "Diff.Files"=w327, "Git.git-api"=w329) -> (w332:T1)
        n129 = call <vilib>:"Add State(s) to Queue__JKI_lib_State_Machine.vi"("State(s) in (\"\")"=w335) -> ("States Out"=w334:string)  [unwired: 14 in]
      }
    }
  }
